vi "TestInitializeLocalLogMultipleSinks_LogEventCaptured.vi"(8 "error in (no error)":errorcluster, 11 "TestCase in":refnum<class "TestMalleableInterface.lvclass">) -> (0 "error out":errorcluster, 3 "TestCase out":refnum<class "TestMalleableInterface.lvclass">)   [LabVIEW 2017, in "TestMalleableInterface.lvclass"]
uses:
  TestMalleableInterface.lvclass
  Source/LVQueue Sink/LVQueue Sink.lvclass/LVQueue Sink.ctl
  Source/Composed Log/LoggerReference/LoggerReference.lvclass/LoggerReference.ctl
  8d299841-f253-422a-a7a1-59edf70c310f.vi
  Source/Composed Log/LoggerReference/Return Aggregate Queues.vi
  Source/Composed Log/LoggerReference/Add Aggregate Log.vi
  8d299841-f253-422a-a7a1-59edf70c310f.vi/c9bb2279-8b7e-4c9d-af08-1e27e8e0bbe5.vi
  Source/Composed Log/LoggerReference/Log.vi
  Source/Composed Log/LoggerReference/Send Add Sink.vi
  Source/Composed Log/LoggerReference/Remove Stale Logs.vi
  Source/LVQueue Sink/LVQueue Sink.lvclass
  C:/CS/Internal/LabVIEW/Logger/Source/Composed Log/Log Sink/Log Sink.lvclass
  Source/Composed Log/Application Logger/Launch Worker Loop.vi
  Source/Composed Log/LoggerReference/Initialize Logger Instance.vi
  Source/Composed Log/LoggerReference/LoggerReference.lvclass
  Source/Composed Log/IErrorFormat/IErrorFormat.lvclass
  Source/Composed Log/Log Sink/Log Sink.lvclass
  <vilib>/addons/_JKI Toolkits/VI Tester/TestCase.llb/TestCase.lvclass
  C:/Program Files (x86)/National Instruments/LabVIEW 2017/vi.lib/addons/_JKI Toolkits/VI Tester/TestCase.llb/TestCase.lvclass
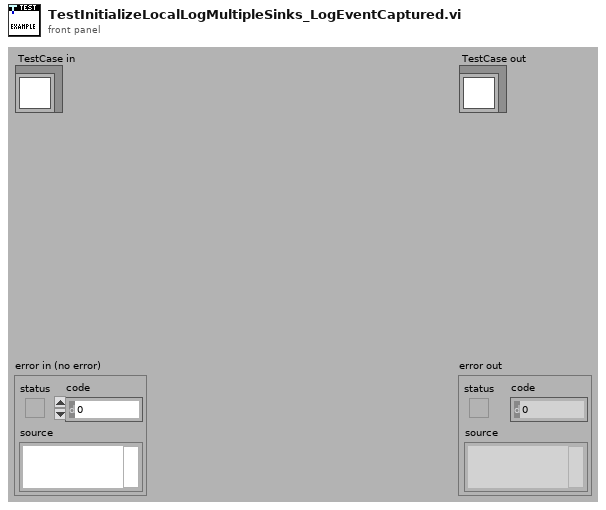
[diagram p1: front panel]
types:
  T1 = typedef "Composed Log.lvlib/Log Packet.ctl" = cluster{"Data To Log":string, "Source":string, "Event Level":T2, "Event Time":timestamp}
  T2 = typedef "Composed Log.lvlib/Log Level.ctl" = enum16{"Debug", "Info", "Warning", "Error", "Critical"}
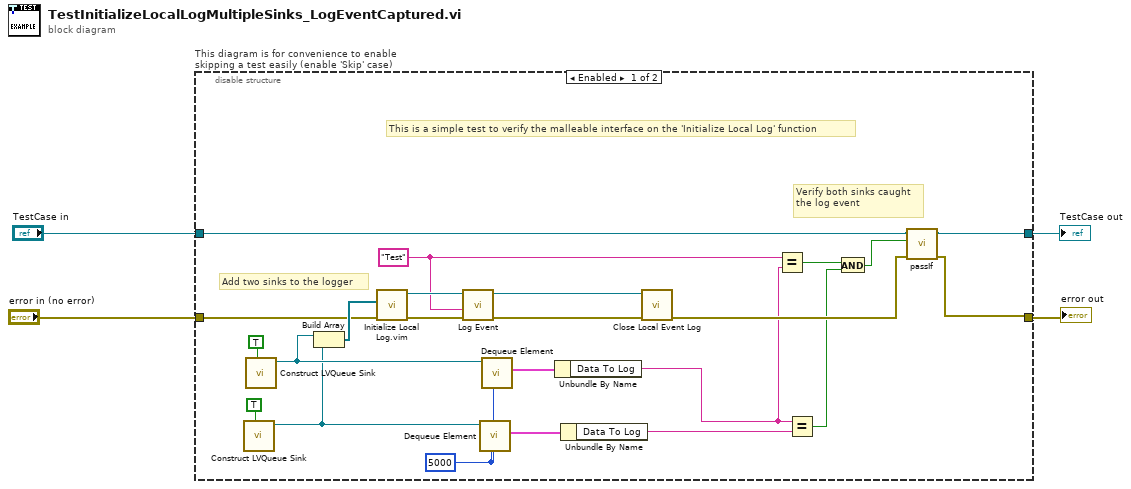
[diagram p0: block diagram]
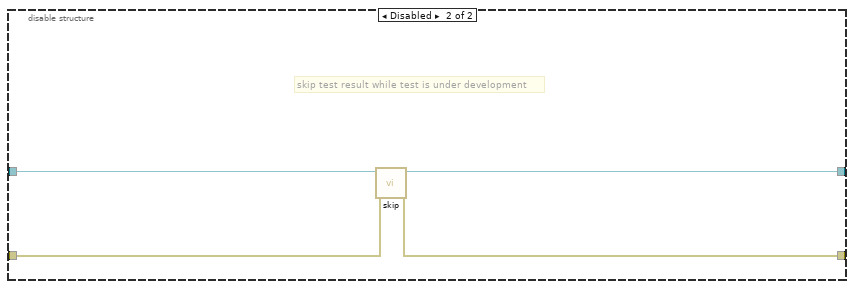
[diagram p2: hidden frame]
diagram:
  n1 = disable-structure "This diagram is for convenience to enable skipping a test easily (enable 'Skip' case)" shown="Enabled" {
    disable-tunnel: "TestCase in" -> [w12 w31]
    disable-tunnel: [w13 w29] -> w1
    disable-tunnel: [w14 w30] -> w3
    disable-tunnel: "error in (no error)" -> [w21 w28]
    frame Enabled {
      w5 = 5000 ("timeout in ms (-1)")
      w10 = "Test" ("SourceID")
      # "This is a simple test to verify the malleable interface on the 'Initialize Local Log' function"
      # "Verify both sinks caught the log event"
      # "Add two sinks to the logger"
      n2 = call "Construct LVQueue Sink.vi"("User Shutdown? (F)"=TRUE) -> ("LVQueue Sink out"=w18:refnum<class "LVQueue Sink.lvclass">)  [unwired: 9 in, 1 out]
      n3 = call "Construct LVQueue Sink.vi"("User Shutdown? (F)"=TRUE) -> ("LVQueue Sink out"=w19:refnum<class "LVQueue Sink.lvclass">)  [unwired: 9 in, 1 out]
      n4 = Build Array(w19, w18) -> (w22:refnum<class "LVQueue Sink.lvclass">[])
      n5 = call "Initialize Local Log.vim"("error in (no error)"=w21, "Startup Sink(s)"=w22) -> ("error out"=w20:errorcluster, "Log Instance Reference"=w24:refnum<class "LoggerReference.lvclass">)  [unwired: 7 in, 1 out]
      n6 = call "Log Event.vi"("error in (no error)"=w20, "Data To Log"=w10, "Log Instance"=w24) -> ("error out"=w26:errorcluster, "Log Instance Out"=w25:refnum<class "LoggerReference.lvclass">)  [unwired: 7 in]
      n7 = call "Dequeue Element.vi"("timeout in ms (-1)"=w5, "LVQueue Sink in"=w18) -> ("Log Packet"=w16:T1)  [unwired: 6 in, 3 out]
      n8 = call "Dequeue Element.vi"("timeout in ms (-1)"=w5, "LVQueue Sink in"=w19) -> ("Log Packet"=w17:T1)  [unwired: 6 in, 3 out]
      n9 = Unbundle By Name(w17) -> ("Data To Log"=w9:string)
      n10 = Unbundle By Name(w16) -> ("Data To Log"=w11:string)
      n11 = call "Close Local Event Log.vi"("error in (no error)"=w26, "Log Instance"=w25) -> ("error out"=w15:errorcluster)  [unwired: 9 in]
      n12 = Equal?(x=w10, y=w9) -> (x = y?=w8:bool)
      n13 = Equal?(x=w9, y=w11) -> (x = y?=w7:bool)
      n14 = And(x=w8, y=w7) -> (x .and. y?=w6:bool)
      n15 = call-dynamic "passIf.vi"("error in (no error)"=w15, "pass"=w6, "TestCase in"=w12) -> ("error out"=w14:errorcluster, "TestCase out"=w13:refnum<class "TestMalleableInterface.lvclass">)  [unwired: 7 in]
    }
    frame Disabled {
      # "skip test result while test is under development"
      n16 = call <vilib>:"skip.vi"("error in (no error)"=w28, "TestCase in"=w31) -> ("error out"=w30:errorcluster, "TestCase out"=w29:refnum<class "TestMalleableInterface.lvclass">)  [unwired: 8 in]
    }
  }
  "error out" <- w3
  "TestCase out" <- w1
